vi "Q1.vi"() -> ()   [LabVIEW 2020]
uses:
  <vilib>/addons/Modulation/Digital/Channel Coding/MT Convolutional Encoder (Rate).vi
  <vilib>/addons/Modulation/Digital/Support/Common/Validators/mod_Validate Bit Stream.vi
  <vilib>/addons/Modulation/Digital/Channel Coding/Convolutional codes/mod_Convolutional encoder.vi
  <vilib>/addons/Modulation/Analog/support/mod_Set Error Source.vi
  <vilib>/addons/Modulation/Digital/Support/Common/Validators/mod_AWGN Validate.vi
  <vilib>/addons/Modulation/Digital/Impairments/subVIs/mod_createSeeds.vi
  <vilib>/addons/Modulation/Digital/Channel Coding/Convolutional codes/subVIs/mod_Generate encoder tap connections.vi
  <vilib>/addons/Modulation/Digital/Channel Coding/Convolutional codes/subVIs/mod_Perform convolutional encoding.vi
  <vilib>/addons/Modulation/Digital/Channel Coding/Block codes/subVIs/mod_Buffer block code info (I8).vi
  <vilib>/addons/Modulation/Digital/Channel Coding/Convolutional codes/subVIs/mod_Generate valid reset (convolutional, I8).vi
  <vilib>/addons/Modulation/Digital/Support/Common/Validators/mod_Validate Samples Per Symbol.vi
  <vilib>/addons/Modulation/Analog/support/Validators/mod_Validate Complex Waveform.vi
  <vilib>/addons/Modulation/Analog/support/Validators/mod_WFErrorHandler.vi
  <vilib>/addons/Modulation/Digital/Channel Coding/Convolutional codes/subVIs/mod_Select known generator matrix.vi
  <vilib>/addons/Modulation/Digital/Support/Common/Validators/mod_Validate Convolutional Encoder prms.vi
  <vilib>/addons/Modulation/Digital/Channel Coding/MT Hamming Encoder (Systematic).vi
  <vilib>/addons/Modulation/Digital/General/MT Generate PSK System Parameters(M).vi
  <vilib>/addons/Modulation/Digital/Support/Common/Validators/mod_Generate Filter Coefficients Validate.vi
  <vilib>/addons/Modulation/Digital/General/subVIs/mod_Generate Filter Coefficients.vi
  <vilib>/addons/Modulation/Digital/General/MT Generate QAM System Parameters(M).vi
  <vilib>/addons/Modulation/Digital/Impairments/Fading Profiles/MT Rayleigh Fading Profile (Jakes).vi
  <vilib>/addons/Modulation/Digital/Impairments/MT Apply Flat Fading Profile.vi
  <vilib>/addons/Modulation/Digital/General/subVIs/mod_Generate Bits PN Sequence.vi
  <vilib>/Analysis/1siggen.llb/Gaussian White Noise (obs 90).vi
  <vilib>/addons/Modulation/Digital/Channel Coding/MT Convolutional Decoder (Viterbi Hard Decision, Rate).vi
  <vilib>/addons/Modulation/Digital/Channel Coding/MT Hamming Decoder (Systematic).vi
  <vilib>/addons/Modulation/niDMT.lvlib
panel:
  in  "Fading (Yes/No)":bool
  in  "Image Path":path
  in  "fading variance":dbl=1.0 format="%.2f"
  in  "(7, 4) Hamming / Convolutional Encoding":bool
  out "modulation type":T1(ring)
  in  "pulse shaping filter (none) 2":T2(ring)
  in  "QPSK / 64-QAM":bool
  out "Received Constellation Graph":T3(graph)
  in  "Eb/N0 (dB)":dbl=10.0 format="%.2f"
  out "Transmit Constellation Graph":T3(graph)
  in  "pulse shaping filter (none)":T2(ring)
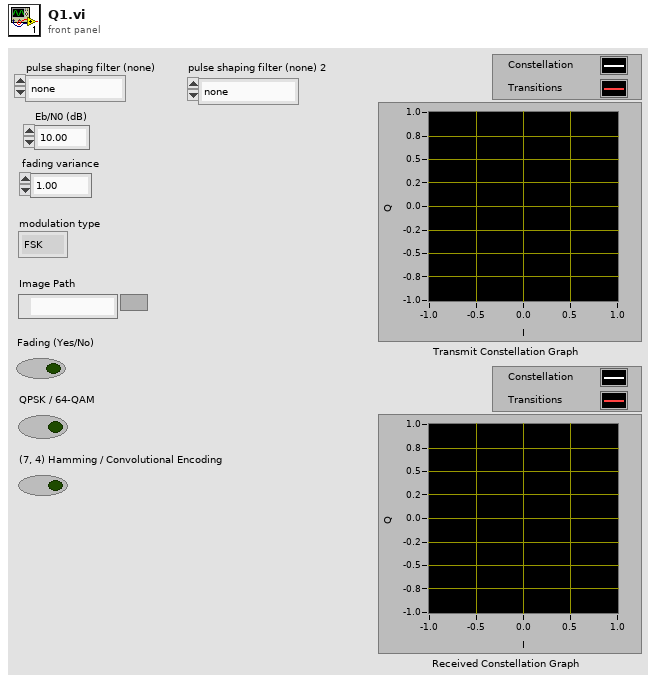
[diagram p1: front panel]
types:
  T1 = enum16{"FSK", "PSK", "QAM", "MSK", "PAM", "ASK", "CPM"}
  T2 = enum16{"none", "Raised Cosine", "Root Raised Cos", "Gaussian"}
  T3 = cluster{"Decimated Array":dbl[], "Decimated Array":dbl[]}[]
  T4 = cluster{"samples per symbol (16)":i32, "symbol map":cdb[], "differential PSK":enum16{"disable", "enable"}, "PSK type":u16}
  T5 = typedef "niAMT.lvlib/Complex Data Waveform.ctl" = cluster{"t0":dbl, "dt":dbl, "Y":cdb[]}
  T6 = cluster{"samples per symbol (16)":i32, "symbol map":cdb[]}
  T7 = cluster{"constellation":dbl[], "oversampled data":dbl[]}[]
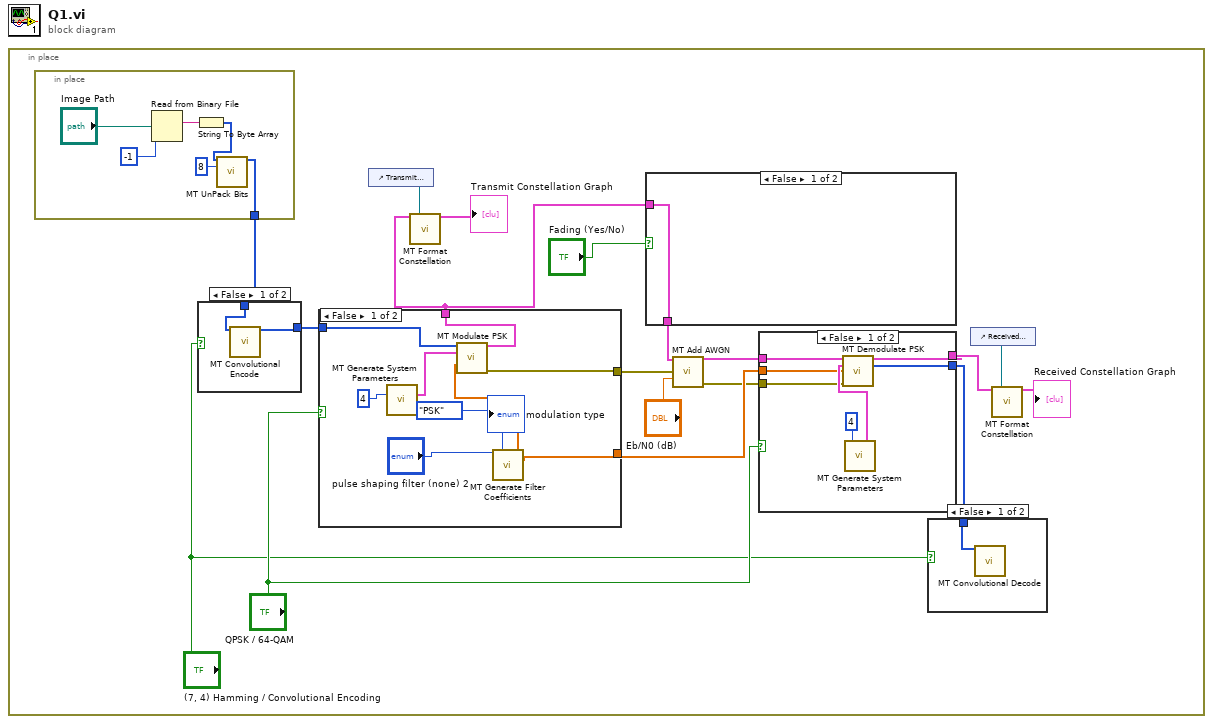
[diagram p0: block diagram]
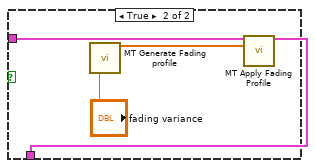
[diagram p2: hidden frame]
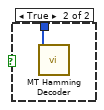
[diagram p3: hidden frame]
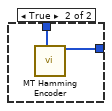
[diagram p4: hidden frame]
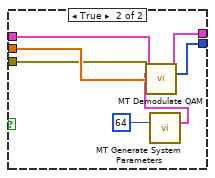
[diagram p5: hidden frame]
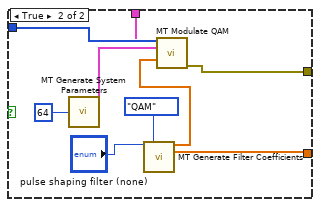
[diagram p6: hidden frame]
diagram:
  n1 = in-place {
    n2 = in-place {
      in-place-border: [w24] -> w3
      n3 = Read from Binary File(10:-1 ("count (1)"), 11:"Image Path") -> (2:w28:string)  [unwired: 4 in, 3 out]
      n4 = String To Byte Array(string=w28) -> (unsigned byte array=w27:u8[])
      n5 = call <vilib>:"MT UnPack Bits.vi"("input integers"=w27, "bits per integer"=8) -> ("output bit stream"=w24:i8[])  [unwired: 12 in, 1 out]
    }
    n6 = case shown="False" "(7, 4) Hamming / Convolutional Encoding" {
      tunnel: w3 -> [w33 w35]
      tunnel: [w32 w34] -> w9
      frame False {
        n7 = call-poly <vilib>:"MT Convolutional Encode.vi"("input bit stream"=w33) -> ("output bit stream"=w32:i8[])  [unwired: 12 in, 2 out]
      }
      frame True {
        n8 = call-poly <vilib>:"MT Hamming Encoder.vi"("input bit stream"=w35) -> ("output bit stream"=w34:i8[])  [unwired: 13 in, 1 out]
      }
    }
    n9 = case shown="False" "QPSK / 64-QAM" {
      tunnel: [w55 w62] -> w5
      tunnel: [w50 w61] -> w16
      tunnel: [w52 w60] -> w14
      tunnel: w9 -> [w57 w63]
      frame False {
        n10 = call-poly <vilib>:"MT Generate System Parameters.vi"("M-PSK (4)"=4) -> ("PSK system parameters"=w58:T4)  [unwired: 12 in, 2 out]
        n11 = call <vilib>:"MT Generate Filter Coefficients.vi"("pulse shaping filter (none)"="pulse shaping filter (none) 2", "modulation type"=T1."PSK") -> ("pulse shaping filter coefficients"=w51:dbl[], "matched filter coefficients"=w52:dbl[])  [unwired: 11 in, 1 out]
        n12 = call <vilib>:"MT Modulate PSK.vi"("input bit stream"=w57, "PSK system parameters"=w58, "pulse shaping filter coefficients"=w51) -> ("output complex waveform"=w55:T5, "error out"=w50:errorcluster)  [unwired: 10 in, 1 out]
      }
      frame True {
        n13 = call-poly <vilib>:"MT Generate System Parameters.vi"("M-QAM (16)"=64) -> ("QAM system parameters"=w67:T6)  [unwired: 12 in, 2 out]
        n14 = call <vilib>:"MT Generate Filter Coefficients.vi"("pulse shaping filter (none)"="pulse shaping filter (none)", "modulation type"=T1."QAM") -> ("pulse shaping filter coefficients"=w66:dbl[], "matched filter coefficients"=w60:dbl[])  [unwired: 11 in, 1 out]
        n15 = call <vilib>:"MT Modulate QAM.vi"("input bit stream"=w63, "QAM system parameters"=w67, "pulse shaping filter coefficients"=w66) -> ("output complex waveform"=w62:T5, "error out"=w61:errorcluster)  [unwired: 10 in, 1 out]
      }
    }
    n16 = control-ref of="Transmit Constellation Graph"() -> (w18:refnum<vi>)
    n17 = call <vilib>:"MT Format Constellation.vi"("waveform"=w5, "constellation reference"=w18) -> ("constellation graph"=→"Transmit Constellation Graph":T7)  [unwired: 3 in, 10 out]
    n18 = case shown="False" "Fading (Yes/No)" {
      tunnel: w5 -> [w19 w21]
      tunnel: [w19 w20] -> w4
      frame False {
      }
      frame True {
        n19 = call-poly <vilib>:"MT Generate Fading profile.vi"("fading variance"="fading variance") -> ("fading profile"=w23:cdb[])  [unwired: 12 in, 2 out]
        n20 = call-poly <vilib>:"MT Apply Fading Profile.vi"("input complex waveform"=w21, "fading profile"=w23) -> ("output complex waveform"=w20:T5)  [unwired: 12 in, 1 out]
      }
    }
    n21 = call <vilib>:"MT Add AWGN.vi"("input complex waveform"=w4, "Eb/N0 (10 dB)"="Eb/N0 (dB)", "error in (no error)"=w16) -> ("output complex waveform"=w6:T5, "error out"=w11:errorcluster)  [unwired: 10 in, 1 out]
    n22 = case shown="False" "QPSK / 64-QAM" {
      tunnel: w14 -> [w37 w49]
      tunnel: w6 -> [w40 w48]
      tunnel: w11 -> [w36 w47]
      tunnel: [w38 w44] -> w10
      tunnel: [w39 w43] -> w7
      frame False {
        n23 = call-poly <vilib>:"MT Generate System Parameters.vi"("M-PSK (4)"=4) -> ("PSK system parameters"=w41:T4)  [unwired: 12 in, 2 out]
        n24 = call <vilib>:"MT Demodulate PSK.vi"("input complex waveform"=w40, "PSK system parameters"=w41, "matched filter coefficients"=w37, "error in (no error)"=w36) -> ("recovered complex waveform"=w39:T5, "output bit stream"=w38:i8[])  [unwired: 7 in, 3 out]
      }
      frame True {
        n25 = call-poly <vilib>:"MT Generate System Parameters.vi"("M-QAM (16)"=64) -> ("QAM system parameters"=w46:T6)  [unwired: 12 in, 2 out]
        n26 = call <vilib>:"MT Demodulate QAM.vi"("input complex waveform"=w48, "QAM system parameters"=w46, "matched filter coefficients"=w49, "error in (no error)"=w47) -> ("recovered complex waveform"=w43:T5, "output bit stream"=w44:i8[])  [unwired: 7 in, 3 out]
      }
    }
    n27 = case shown="False" "(7, 4) Hamming / Convolutional Encoding" {
      tunnel: w10 -> [w30 w31]
      frame False {
        n28 = call-poly <vilib>:"MT Convolutional Decode.vi"("input bit stream"=w30) -> ()  [unwired: 12 in, 3 out]
      }
      frame True {
        n29 = call-poly <vilib>:"MT Hamming Decoder.vi"("input bit stream"=w31) -> ()  [unwired: 13 in, 2 out]
      }
    }
    n30 = control-ref of="Received Constellation Graph"() -> (w13:refnum<vi>)
    n31 = call <vilib>:"MT Format Constellation.vi"("waveform"=w7, "constellation reference"=w13) -> ("constellation graph"=→"Received Constellation Graph":T7)  [unwired: 3 in, 10 out]
  }
